vi "Dequeue Transport Element.vi"(8 "error in (no error)":errorcluster, 9 "Timeout In ms (-1)":i32=-1, 11 "QueueTransport":refnum<class "QueueTransport.lvclass">) -> (0 "error out":errorcluster, 1 "Publication Time":timestamp, 2 "Data":variant, 4 "Data Lost?":bool)   [LabVIEW 2020, in "QueueTransport.lvclass"]
uses:
  <vilib>/gpm_packages/@cs/transport/Source/Concrete/QueueTransport/QueueTransport.lvclass
  <vilib>/gpm_packages/@cs/transport/Source/Concrete/QueueTransport/QueueTransport.lvclass/QueueTransport.ctl
  <vilib>/Utility/error.llb/Error Cluster From Error Code.vi
  <vilib>/ErrorRing/Error Ring.xnode
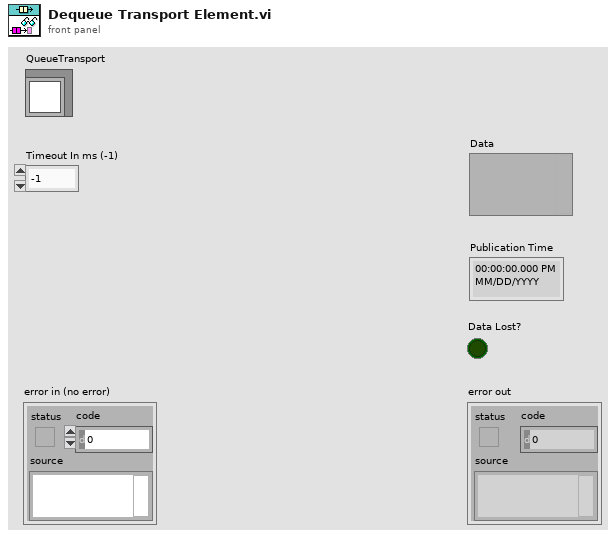
[diagram p1: front panel]
types:
  T1 = cluster{"Data":variant, "Publication Time":timestamp}
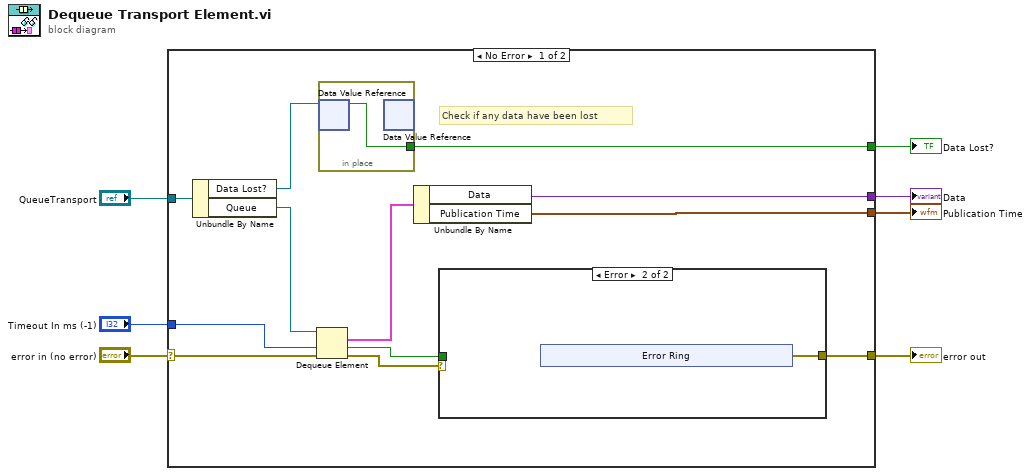
[diagram p0: block diagram]
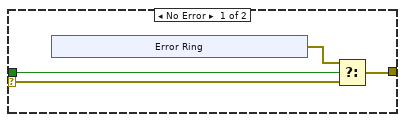
[diagram p2: hidden frame]
diagram:
  n1 = case shown="No Error" "error in (no error)" {
    selector: "error in (no error)" -> [w19 w36]
    tunnel: "QueueTransport" -> [w18 _]
    tunnel: "Timeout In ms (-1)" -> [w17 _]
    tunnel: [w15 _] -> w4
    tunnel: [w14 _] -> w3
    tunnel: [w12 w36] -> w2
    tunnel: [w8 _] -> w1
    frame No Error {
      # "Check if any data have been lost"
      n2 = Unbundle By Name(w18) -> ("Data Lost?"=w9:refnum<data-value>, "Queue"=w13:refnum<queue>)
      n3 = Dequeue Element(queue=w13, timeout in ms (-1)=w17, error in (no error)=w19) -> (element=w16:T1, timed out?=w11:bool, error out=w10:errorcluster)  [unwired: 1 out]
      n4 = in-place {
        in-place-border: [w20] -> w8
        n5 = in-place-dvr #1(w9) -> (w20:bool)  [unwired: 1 out]
        n6 = in-place-dvr #1() -> ()  [unwired: 1 in, 2 out]
      }
      n7 = Unbundle By Name(w16) -> ("Data"=w15:variant, "Publication Time"=w14:timestamp)
      n8 = case shown="Error" w10 {
        selector: w10 -> [w22 _]
        tunnel: [w24 w30] -> w12
        tunnel: w11 -> [w23 _]
        frame No Error {
          n9 = xnode "Error Ring"() -> ("error out"=w21:errorcluster)
          n10 = Select(t=w21, s=w23, f=w22) -> (s? t:f=w24:errorcluster)
        }
        frame Error {
          n11 = xnode "Error Ring"() -> ("error out"=w30:errorcluster)
        }
      }
    }
    frame Error {
    }
  }
  "error out" <- w2
  "Data" <- w4
  "Publication Time" <- w3
  "Data Lost?" <- w1
